vi "Filter Error Codes (Array)__ogtk.vi"(4 "Upstream Error (optional)":errorcluster, 8 "Error In":errorcluster, 10 "Error Codes to Filter":i32[](array[numeric])) -> (0 "Error Out":errorcluster, 1 "Error Filtered?":bool, 2 "Filtered Error Details":T1)   [LabVIEW 2016]
doc: "Filters <b>Error In</b> if matches <b>Error Code to Filter</b>. An <b>Upstream Error</b> can be optionally merged with the resulting filtered error."
uses:
  <userlib>/_OpenG.lib/error/error.llb/Filtered Error Details - Cluster__ogtk.ctl
panel:
  # "Please visit http://www.OpenG.org to learn about the\nOpen Source LabVIEW software movement.\n\nNOTICE -- YOU MUST LEAVE THIS NOTICE IN PLACE.  PER THE TERMS OF THE LICENSE BELOW, YOU MAY SUBLICENSE THIS SOFTWARE \nIN ANY WAY THAT DOES NOT CONFLICT WITH THIS LICENSE.\n\n### BSD License (http://www.opensource.org/licenses/bsd-license.php) Begin ###\n \nCopyright (c) 2011, JKI <info@jki.net>\nCopyright (c) 2011, Jonathon Green <jg@jgcode.net>\n\nAll rights reserved.\n\nRedistribution and use in source and binary forms, with or without modification, are permitted provided that the following conditions are met:\n\n    * Redistributions of source code must retain the above copyright notice, this list of conditions and the following disclaimer.\n    * Redistributions in binary form must reproduce the above copyright notice, this list of conditions and the following disclaimer in the \n       documentation and/or other materials provided with the distribution.\n    * Neither the name of SciWare, James Kring, Inc., nor the names of its contributors may be used to endorse or promote products derived \n       from this software without specific prior written permission.\n\nTHIS SOFTWARE IS PROVIDED BY THE COPYRIGHT HOLDERS AND CONTRIBUTORS \"AS IS\" AND ANY EXPRESS OR IMPLIED WARRANTIES, \nINCLUDING, BUT NOT LIMITED TO, THE IMPLIED WARRANTIES OF MERCHANTABILITY AND FITNESS FOR A PARTICULAR PURPOSE ARE \nDISCLAIMED. IN NO EVENT SHALL THE COPYRIGHT OWNER OR CONTRIBUTORS BE LIABLE FOR ANY DIRECT, INDIRECT, INCIDENTAL,\n SPECIAL, EXEMPLARY, OR CONSEQUENTIAL DAMAGES (INCLUDING, BUT NOT LIMITED TO, PROCUREMENT OF SUBSTITUTE GOODS OR \nSERVICES; LOSS OF USE, DATA, OR PROFITS; OR BUSINESS INTERRUPTION) HOWEVER CAUSED AND ON ANY THEORY OF LIABILITY, \nWHETHER IN CONTRACT, STRICT LIABILITY, OR TORT (INCLUDING NEGLIGENCE OR OTHERWISE) ARISING IN ANY WAY OUT OF THE USE \nOF THIS SOFTWARE, EVEN IF ADVISED OF THE POSSIBILITY OF SUCH DAMAGE.\n\n### BSD License End ###"
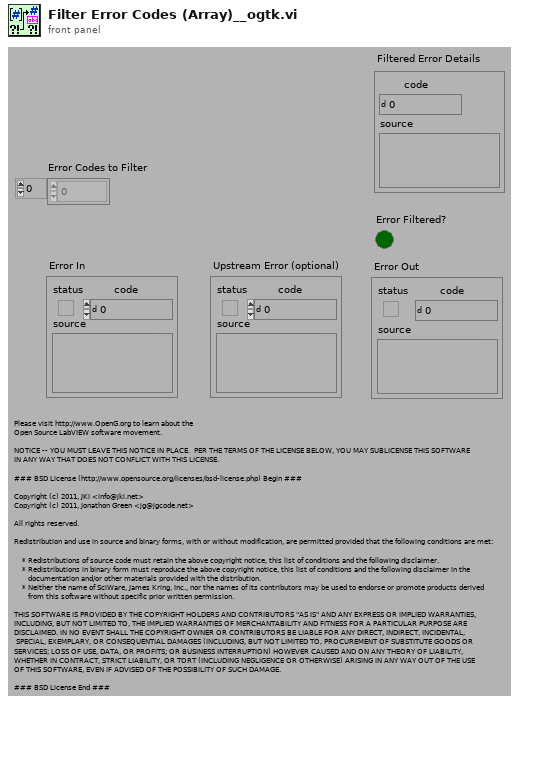
[diagram p1: front panel]
types:
  T1 = typedef "Filtered Error Details - Cluster__ogtk.ctl" = cluster{"code":i32, "source":string}
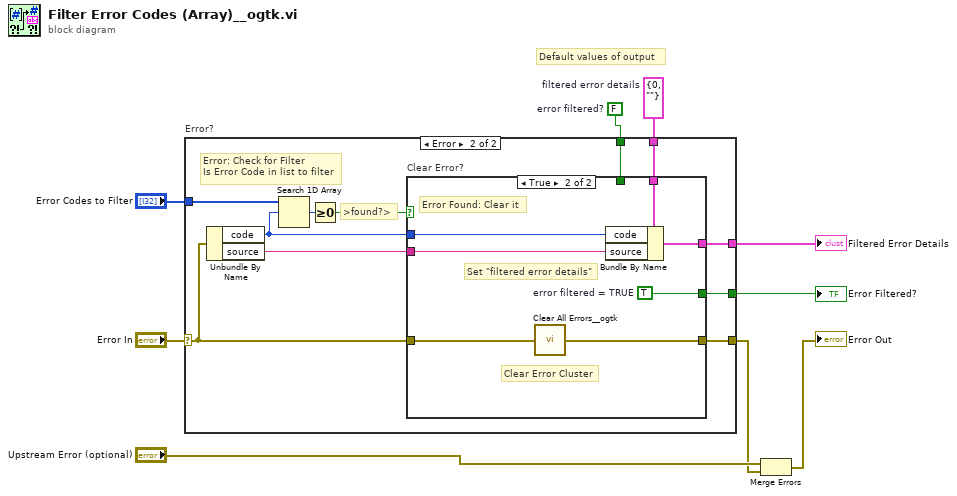
[diagram p0: block diagram]
diagram:
  w4 = FALSE  # error filtered?
  w5 = T1 {"code"=0, "source"=""}  # filtered error details
  # "Default values of output"
  n1 = case "Error?" shown="Error" "Error In" {
    selector: "Error In" -> [w12 w20]
    tunnel: [w12 w19] -> w1
    tunnel: "Error Codes to Filter" -> [_ w18]
    tunnel: [w10 w22] -> w7
    tunnel: [w11 w21] -> w6
    tunnel: w5 -> [w10 w14]
    tunnel: w4 -> [w11 w13]
    frame No Error {
      # "No Error: Do nothing"
    }
    frame Error {
      # "Error: Check for Filter\nIs Error Code in list to filter"
      # ">found?>"
      n2 = Unbundle By Name(w20) -> ("code"=w17:i32, "source"=w23:string)
      n3 = Search 1D Array(1D array=w18, element=w17) -> (index of element=w16:i32)  [unwired: 1 in]
      n4 = Greater Or Equal To 0?(x=w16) -> (x >= 0?=w15:bool)
      n5 = case "Clear Error?" shown="True" w15 {
        tunnel: w23 -> [_ w33]
        tunnel: [w25 w32] -> w22
        tunnel: [w24 w29] -> w21
        tunnel: w17 -> [_ w31]
        tunnel: w20 -> [w26 w28]
        tunnel: [w26 w27] -> w19
        tunnel: w14 -> [w25 w30]
        tunnel: w13 -> [w24 _]
        frame False {
          # "Error Not Found: Do nothing (use default outputs)"
        }
        frame True {
          w29 = TRUE  # error filtered = TRUE
          # "Set \"filtered error details\""
          # "Clear Error Cluster"
          # "Error Found: Clear it"
          n6 = call <userlib>:"Clear All Errors__ogtk.vi"("Error In"=w28) -> ("Error Out"=w27:errorcluster)  [unwired: 3 in]
          n7 = Bundle By Name(cluster=w30, "code"=w31, "source"=w33) -> (w32:T1)
        }
      }
    }
  }
  "Filtered Error Details" <- w7
  "Error Filtered?" <- w6
  n8 = Merge Errors("Upstream Error (optional)", w1) -> (→"Error Out":errorcluster)
